vi "1WIRE_RESET_multi.vi"(8 "error in":errorcluster, 11 "FPGA I/O In":refnum<k21>="DS_WIRE") -> (0 "error out":errorcluster, 1 "0 = Device Present / 1=no":bool)   [LabVIEW 2016]
doc: "This VI is created by Vincent Claes for FPDA-1 more information on http://pwo.fpga.be\n\nvincent.claes@xios.be\nclaesvincent@gmail.com\n\nhttp://www.linkedin.com/in/vincentclaes"
uses:
  <vilib>/rvi/Emulation/niFpgaSctlEmulationGetInTimedLoop.vi
  <vilib>/rvi/Emulation/niFpgaProcessEmulError.vi
  <vilib>/rvi/eio/common/nirviEmuTemplateMethod_errors.vi
  <vilib>/eio/EIOMethodNode/EIOMethodNode.xnode
  <vilib>/eio/EIONode/EIONode.xnode
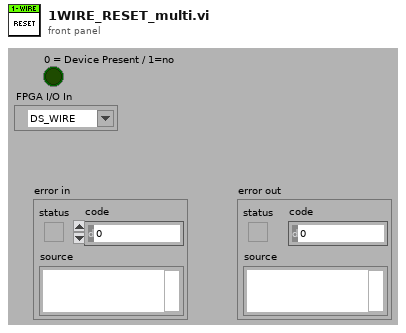
[diagram p1: front panel]
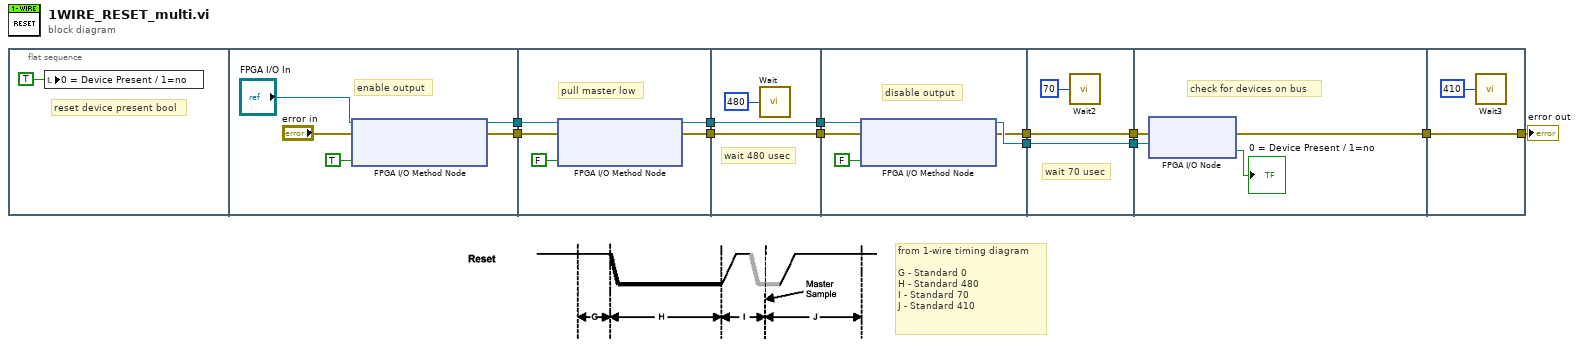
[diagram p0: block diagram]
diagram:
  # "from 1-wire timing diagram\n\nG - Standard 0\nH - Standard 480\nI - Standard 70\nJ - Standard 410"
  n1 = flat-sequence {
    tunnel: [w17] -> w12
    tunnel: [w16] -> w11
    tunnel: w12 -> [w23]
    tunnel: w11 -> [w22]
    tunnel: [w21] -> w3
    tunnel: [w20] -> w2
    tunnel: [w25] -> w4
    tunnel: w3 -> [w25]
    tunnel: w2 -> [w24]
    tunnel: [w24] -> w1
    tunnel: [w30] -> w10
    tunnel: [w29] -> w9
    tunnel: w4 -> [w28]
    tunnel: w1 -> [w27]
    tunnel: [w33] -> w8
    tunnel: w10 -> [w33]
    tunnel: w9 -> [w32]
    tunnel: [w32] -> w7
    tunnel: w8 -> [w37]
    tunnel: w7 -> [w36]
    tunnel: [w35] -> w6
    tunnel: w6 -> [w39]
    tunnel: [w39] -> w5
    frame #0 {
      # "reset device present bool"
      n2 = local write "0 = Device Present / 1=no"(TRUE ("0 = Device Present / 1=no")) -> ()
    }
    frame #1 {
      # "enable output"
      n3 = xnode "FPGA I/O Method Node"("error in"="error in", "FPGA I/O In"="FPGA I/O In", "Enable"=TRUE ("Data")) -> ("error out"=w16:errorcluster, "FPGA I/O Out"=w17:refnum<k21>)
    }
    frame #2 {
      # "pull master low"
      n4 = xnode "FPGA I/O Method Node"("error in"=w22, "FPGA I/O In"=w23, "Data"=FALSE ("FX2_IO1_J1_0")) -> ("error out"=w20:errorcluster, "FPGA I/O Out"=w21:refnum<k21>)
    }
    frame #3 {
      # "wait 480 usec"
      n5 = call "Wait"("Count(uSec)"=u32 480) -> ()  [unwired: 1 out]
    }
    frame #4 {
      # "disable output"
      n6 = xnode "FPGA I/O Method Node"("error in"=w27, "FPGA I/O In"=w28, "Enable"=FALSE ("Data")) -> ("error out"=w29:errorcluster, "FPGA I/O Out"=w30:refnum<k21>)
    }
    frame #5 {
      # "wait 70 usec"
      n7 = call "Wait2"("Count(uSec)"=u32 70) -> ()  [unwired: 1 out]
    }
    frame #6 {
      # "check for devices on bus"
      n8 = xnode "FPGA I/O Node"("error in"=w36, "FPGA I/O In"=w37) -> ("error out"=w35:errorcluster, "I/O Item"=→"0 = Device Present / 1=no":bool)  [unwired: 1 out]
    }
    frame #7 {
      n9 = call "Wait3"("Count(uSec)"=u32 410) -> ()  [unwired: 1 out]
    }
  }
  "error out" <- w5
